vi "Source Set Level.vi"(6 "DC current [A]":dbl, 8 "error in":errorcluster, 9 "current [A]":dbl, 10 "f [Hz]":dbl, 11 "src in":T1={"type"=enum."Tektronix AFG3101C", "afg"={"VISA"="", "const"=0.0, "gen DC"=FALSE, "ext ref"=FALSE}, "cDAQ dds"={"device"="", "channels"=[], "mclk source"="", "mclk [Hz]"=0.0, "fs [Hz]"=0.0, "block [s]"=0.0, "buf [s]"=0.0, "task"="", "cmd queue"=refnum, "proc ref"=refnum, "smpl clock out"="/cDAQ3/PFI0", "export smpl clock"=FALSE, "DC ofs [V]"=[], "timebase source"="", "timebase mode"=enum."Local"}, "gain [V/A]"=1.0, "F5xxx session"={"VISA"="", "mode"=enum."AC voltage", "Earth on"=FALSE, "Ext ref lock"=FALSE}} {"cDAQ dds"."channels" min=0 step=1}) -> (0 "error out":errorcluster, 3 "src out":T1={"type"=enum."Tektronix AFG3101C", "afg"={"VISA"="", "const"=0.0, "gen DC"=FALSE, "ext ref"=FALSE}, "cDAQ dds"={"device"="", "channels"=[], "mclk source"="", "mclk [Hz]"=0.0, "fs [Hz]"=0.0, "block [s]"=0.0, "buf [s]"=0.0, "task"="", "cmd queue"=refnum, "proc ref"=refnum, "smpl clock out"="/cDAQ3/PFI0", "export smpl clock"=FALSE, "DC ofs [V]"=[], "timebase source"="", "timebase mode"=enum."Local"}, "gain [V/A]"=1.0, "F5xxx session"={"VISA"="", "mode"=enum."AC voltage", "Earth on"=FALSE, "Ext ref lock"=FALSE}} {"cDAQ dds"."channels" min=0 step=1})   [LabVIEW 2013]
doc: "Set source output level."
uses:
  Source Session.ctl
  Source Type.ctl
  drivers/AFG3101C/AFG3101C Session.ctl
  drivers/cDAQ DDS/cDAQ DDS Session.ctl
  drivers/cDAQ DDS/cDAQ DDS Setup.ctl
  drivers/cDAQ DDS/cDAQ DDS Timebase Mode.ctl
  drivers/Fluke 5XXX/top_lev/F5xxx_session.ctl
  drivers/Fluke 5XXX/top_lev/F5xxx_output_mode.ctl
  drivers/AFG3101C/Tektronix AFG 3000 Series.lvlib
  <vilib>/Utility/error.llb/Error Cluster From Error Code.vi
  <vilib>/ErrorRing/Error Ring.xnode
  drivers/Fluke 5XXX/Fluke 5XXX Series Multicalibrators.lvlib
  drivers/Agilent 33XXX Series/Agilent 33XXX Series.lvlib
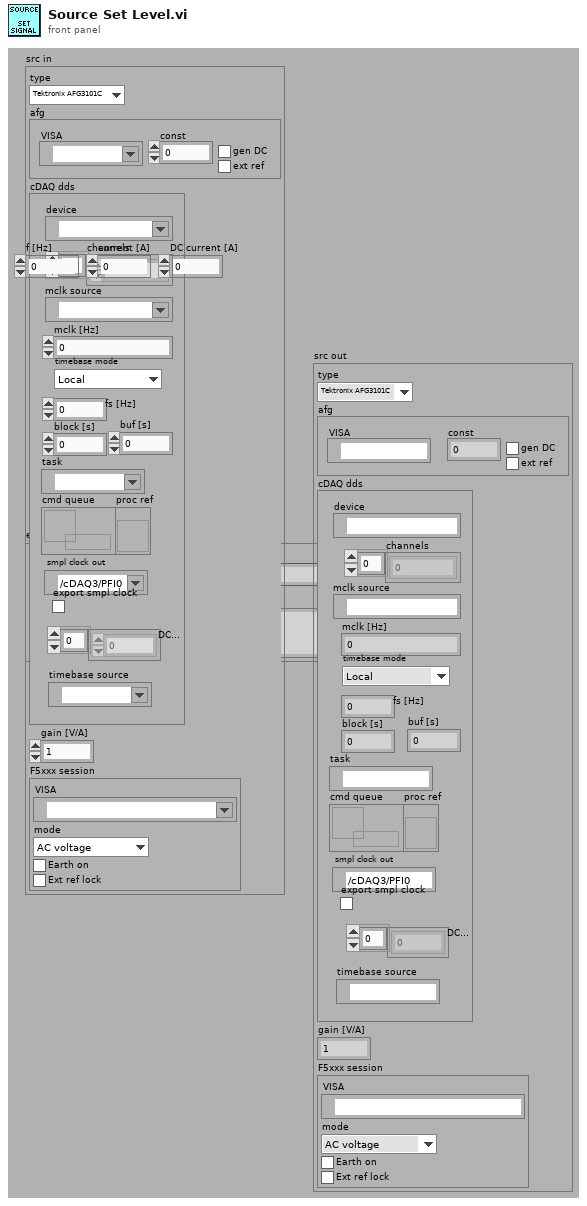
[diagram p1: front panel]
types:
  T1 = typedef "Source Session.ctl" = cluster{"type":T2, "afg":T3, "cDAQ dds":T4, "gain [V/A]":dbl, "F5xxx session":T6}
  T2 = typedef "Source Type.ctl" = enum16{"Tektronix AFG3101C", "cDAQ DAC", "Fluke 5xxx", "Agilent 33120A", "dummy"}
  T3 = typedef "AFG3101C Session.ctl" = cluster{"VISA":refnum<visa-resource-name>, "const":dbl, "gen DC":bool, "ext ref":bool}
  T4 = typedef "cDAQ DDS Session.ctl" = cluster{"device":tag, "channels":i32[], "mclk source":tag, "mclk [Hz]":dbl, "fs [Hz]":dbl, "block [s]":dbl, "buf [s]":dbl, "task":refnum<k21>, "cmd queue":refnum<queue>, "proc ref":refnum<vi>, "smpl clock out":tag, "export smpl clock":bool, "DC ofs [V]":dbl[], "timebase source":tag, "timebase mode":T5}
  T5 = typedef "cDAQ DDS Timebase Mode.ctl" = enum16{"Local", "Take from ADC (e.g. NI 9238)", "Other source"}
  T6 = typedef "F5xxx_session.ctl" = cluster{"VISA":refnum<visa-resource-name>, "mode":T7, "Earth on":bool, "Ext ref lock":bool}
  T7 = typedef "F5xxx_output_mode.ctl" = enum16{"AC voltage", "AC current"}
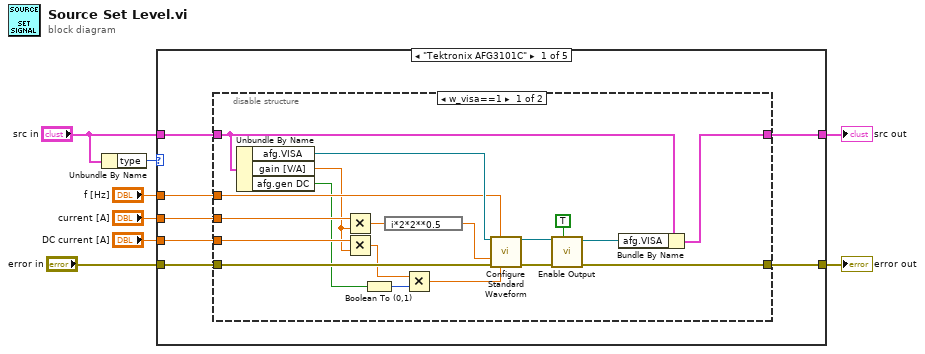
[diagram p0: block diagram]
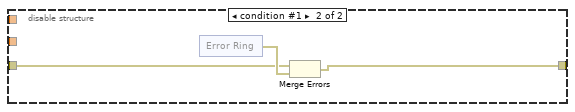
[diagram p2: hidden frame]
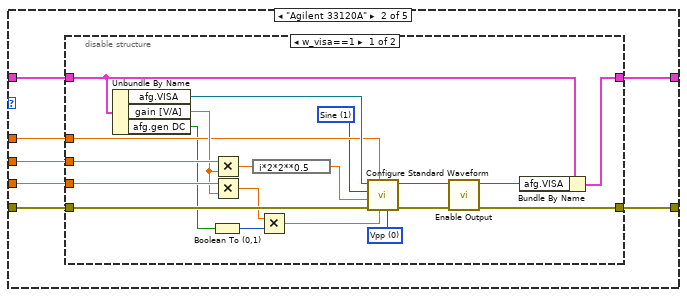
[diagram p3: hidden frame]
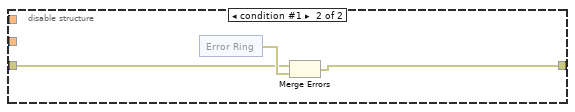
[diagram p4: hidden frame]
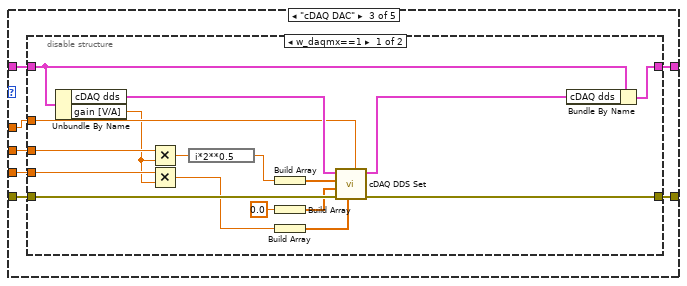
[diagram p5: hidden frame]
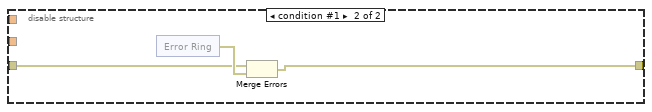
[diagram p6: hidden frame]
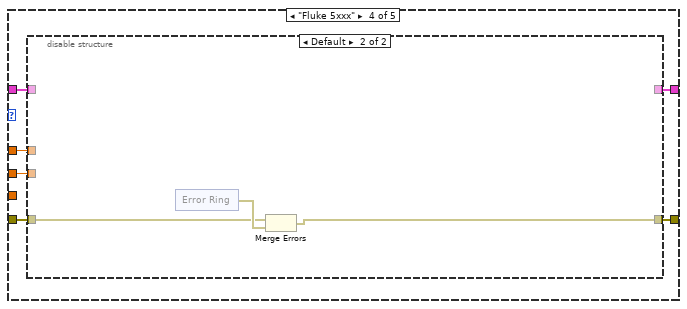
[diagram p7: hidden frame]
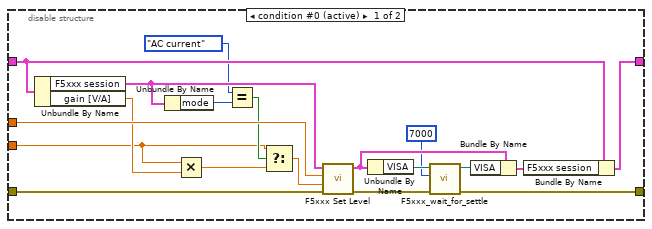
[diagram p8: hidden frame]
diagram:
  n1 = Unbundle By Name("src in") -> ("type"=w7:T2)
  n2 = case shown="\"Tektronix AFG3101C\"" w7 {
    tunnel: "src in" -> [w15 w49 w83 w114 w144]
    tunnel: "error in" -> [w13 w47 w84 w115 w143]
    tunnel: [w9 w43 w81 w112 w143] -> w5
    tunnel: [w14 w48 w82 w113 w144] -> w4
    tunnel: "f [Hz]" -> [w12 w46 w80 w111 _]
    tunnel: "current [A]" -> [w11 w45 w79 w110 _]
    tunnel: "DC current [A]" -> [w10 w44 w78 _ _]
    frame "Tektronix AFG3101C" {
      n3 = disable-structure shown="w_visa==1" {
        disable-tunnel: w15 -> [w34 _]
        disable-tunnel: [w33 _] -> w14
        disable-tunnel: w13 -> [w32 w36]
        disable-tunnel: w12 -> [w30 _]
        disable-tunnel: w11 -> [w29 _]
        disable-tunnel: w10 -> [w27 _]
        disable-tunnel: [w21 w35] -> w9
        frame condition #0 (active) {
          n4 = Unbundle By Name(w34) -> ("afg.VISA"=w31:refnum<visa-resource-name>, "gain [V/A]"=w26:dbl, "afg.gen DC"=w16:bool)
          n5 = Multiply(x=w29, y=w26) -> (x*y=w28:dbl)
          n6 = Multiply(x=w27, y=w26) -> (x*y=w19:dbl)
          n7 = Boolean To (0,1)(Boolean=w16) -> (0, 1=w17:i16)
          n8 = expression code="i*2*2**0.5"(w28) -> (w25:dbl)
          n9 = Multiply(x=w19, y=w17) -> (x*y=w18:dbl)
          n10 = call "Configure Standard Waveform.vi"("VISA resource name"=w31, "Frequency (1000 Hz)"=w30, "Amplitude (1 Vpp)"=w25, "error in (no error)"=w32, "DC Offset (0.00 V)"=w18) -> ("VISA resource name out"=w23:refnum<visa-resource-name>, "error out"=w24:errorcluster)  [unwired: 9 in]
          n11 = call "Enable Output.vi"("Enable Output (T: Enable)"=TRUE, "error in (no error)"=w24, "VISA resource name"=w23) -> ("error out"=w21:errorcluster, "VISA resource name out"=w22:refnum<visa-resource-name>)  [unwired: 7 in]
          n12 = Bundle By Name(cluster=w34, "afg.VISA"=w22) -> (w33:T1)
        }
        frame condition #1 {
          n13 = xnode "Error Ring"() -> ("error out"=w37:errorcluster)
          n14 = Merge Errors(w36, w37) -> (w35:errorcluster)
        }
      }
    }
    frame "Agilent 33120A" {
      n15 = disable-structure shown="w_visa==1" {
        disable-tunnel: w49 -> [w69 _]
        disable-tunnel: [w68 _] -> w48
        disable-tunnel: w47 -> [w61 w71]
        disable-tunnel: w46 -> [w59 _]
        disable-tunnel: w45 -> [w67 _]
        disable-tunnel: w44 -> [w65 _]
        disable-tunnel: [w63 w70] -> w43
        frame condition #0 (active) {
          w54 = u16 0 items=["Vpp", "Vrms", "dB"] ("Unit (0: Vpp)")
          w58 = u16 1 items=["DC", "Sine", "Square", "Triangle", "Ramp", "Pulse", "Noise", "Sinc", "Negative Ramp", "Exponential Rise", "Exponential Fall", "Cardiac"] ("Waveform Function (1: Sine)")
          n16 = Unbundle By Name(w69) -> ("afg.VISA"=w60:refnum<visa-resource-name>, "gain [V/A]"=w64:dbl, "afg.gen DC"=w50:bool)
          n17 = Boolean To (0,1)(Boolean=w50) -> (0, 1=w51:i16)
          n18 = Multiply(x=w67, y=w64) -> (x*y=w66:dbl)
          n19 = Multiply(x=w65, y=w64) -> (x*y=w53:dbl)
          n20 = expression code="i*2*2**0.5"(w66) -> (w57:dbl)
          n21 = Multiply(x=w53, y=w51) -> (x*y=w52:dbl)
          n22 = call "Configure Standard Waveform.vi"("Unit (0: Vpp)"=w54, "DC Offset (0.00 V)"=w52, "Frequency (1000 Hz)"=w59, "error in (no error)"=w61, "Amplitude (1)"=w57, "Waveform Function (1: Sine)"=w58, "VISA resource name"=w60) -> ("error out"=w56:errorcluster, "VISA resource name out"=w55:refnum<visa-resource-name>)  [unwired: 3 in]
          n23 = call "Enable Output.vi"("error in (no error)"=w56, "VISA resource name"=w55) -> ("error out"=w63:errorcluster, "VISA resource name out"=w62:refnum<visa-resource-name>)  [unwired: 8 in]
          n24 = Bundle By Name(cluster=w69, "afg.VISA"=w62) -> (w68:T1)
        }
        frame condition #1 {
          n25 = xnode "Error Ring"() -> ("error out"=w72:errorcluster)
          n26 = Merge Errors(w71, w72) -> (w70:errorcluster)
        }
      }
    }
    frame "cDAQ DAC" {
      n27 = disable-structure shown="w_daqmx==1" {
        disable-tunnel: w84 -> [w101 w103]
        disable-tunnel: w83 -> [w99 _]
        disable-tunnel: [w97 _] -> w82
        disable-tunnel: [w96 w102] -> w81
        disable-tunnel: w80 -> [w95 _]
        disable-tunnel: w79 -> [w92 _]
        disable-tunnel: w78 -> [w91 _]
        frame condition #0 (active) {
          n28 = Unbundle By Name(w99) -> ("cDAQ dds"=w100:T4, "gain [V/A]"=w87:dbl)
          n29 = Multiply(x=w92, y=w87) -> (x*y=w94:dbl)
          n30 = Multiply(x=w91, y=w87) -> (x*y=w86:dbl)
          n31 = expression code="i*2**0.5"(w94) -> (w93:dbl)
          n32 = Build Array(w93) -> (w90:dbl[])
          n33 = Build Array(0.0) -> (w89:dbl[])
          n34 = Build Array(w86) -> (w85:dbl[])
          n35 = call "cDAQ DDS Set.vi"("common f [Hz]"=w95, "ofs [V]"=w85, "error in"=w101, "ph [rad]"=w89, "A [V]"=w90, "cDAQ dds"=w100) -> ("error out"=w96:errorcluster, "cDAQ dds out"=w98:T4)  [unwired: 4 in]
          n36 = Bundle By Name(cluster=w99, "cDAQ dds"=w98) -> (w97:T1)
        }
        frame condition #1 {
          n37 = xnode "Error Ring"() -> ("error out"=w104:errorcluster)
          n38 = Merge Errors(w103, w104) -> (w102:errorcluster)
        }
      }
    }
    frame "Fluke 5xxx" {
      n39 = disable-structure shown="Default" {
        disable-tunnel: w115 -> [w134 w136]
        disable-tunnel: w114 -> [w133 _]
        disable-tunnel: [w132 _] -> w113
        disable-tunnel: [w117 w135] -> w112
        disable-tunnel: w111 -> [w131 _]
        disable-tunnel: w110 -> [w124 _]
        frame condition #0 (active) {
          n40 = Unbundle By Name(w133) -> ("F5xxx session"=w129:T6, "gain [V/A]"=w130:dbl)
          n41 = Unbundle By Name(w129) -> ("mode"=w128:T7)
          n42 = Multiply(x=w124, y=w130) -> (x*y=w123:dbl)
          n43 = Equal?(x=F5xxx_output_mode."AC current", y=w128) -> (x = y?=w126:bool)
          n44 = Select(t=w124, s=w126, f=w123) -> (s? t:f=w125:dbl)
          n45 = call "F5xxx Set Level.vi"("error in (no error)"=w134, "level [V/A]"=w125, "f [Hz]"=w131, "session in"=w129) -> ("error out"=w122:errorcluster, "session out"=w120:T6)  [unwired: 6 in]
          n46 = Unbundle By Name(w120) -> ("VISA"=w121:refnum<visa-resource-name>)
          n47 = call "F5xxx_wait_for_settle.vi"("error in (no error)"=w122, "timeout [ms]"=u32 7000, "VISA Refnum in"=w121) -> ("error out"=w117:errorcluster, "VISA Refnum out"=w119:refnum<visa-resource-name>)  [unwired: 6 in, 1 out]
          n48 = Bundle By Name(cluster=w120, "VISA"=w119) -> (w118:T6)
          n49 = Bundle By Name(cluster=w133, "F5xxx session"=w118) -> (w132:T1)
        }
        frame condition #1 {
          n50 = xnode "Error Ring"() -> ("error out"=w137:errorcluster)
          n51 = Merge Errors(w136, w137) -> (w135:errorcluster)
        }
      }
    }
    frame "dummy", Default {
    }
  }
  "error out" <- w5
  "src out" <- w4
